vi "Test Top State.vi"() -> ()   [LabVIEW 2020]
uses:
  TDefs/State.ctl
  TDefs/States.ctl
  StateMachine.lvlib
panel:
  out "Next States out":T1
  out "Next State":T2
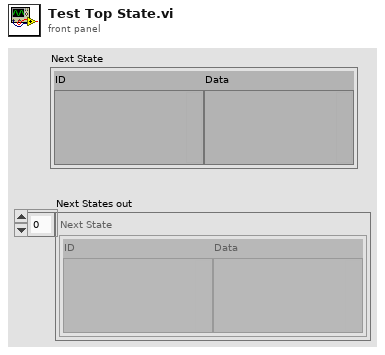
[diagram p1: front panel]
types:
  T1 = typedef "StateMachine.lvlib/States.ctl" = T2[]
  T2 = typedef "StateMachine.lvlib/State.ctl" = cluster{"ID":variant, "Data":variant}
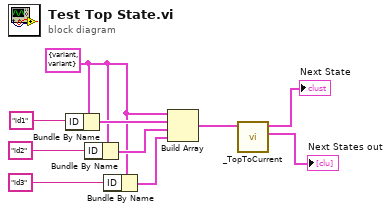
[diagram p0: block diagram]
diagram:
  w1 = T2 {"ID"=variant, "Data"=variant} ("Next State")
  n1 = Bundle By Name(cluster=w1, "ID"="id1") -> (w10:T2)
  n2 = Bundle By Name(cluster=w1, "ID"="id2") -> (w8:T2)
  n3 = Bundle By Name(cluster=w1, "ID"="id3") -> (w6:T2)
  n4 = Build Array(w1, w10, w8, w6) -> (w4:T2[])
  n5 = call "_TopToCurrent.vi"("Next States in"=w4) -> ("Next States out"=→"Next States out":T1, "Next State"=→"Next State":T2)  [unwired: 9 in]
